vi "Xboxinterface_86.vi"() -> (2 "R Thumb":i32(slide) scale=-32768.0..32768.0)   [LabVIEW 2020]
uses:
  <vilib>/robotics/Controls/Compass Indicator/Compass Indicator.xctl
  08dc6dd9-20da-488d-be37-67a715477d84.vi
  <vilib>/Utility/inputDevices.llb/joystickAcquire.vi
  <vilib>/Utility/inputDevices.llb/closeJoystick.vi
panel:
  out "100%":bool
  out "80%":bool
  out "Analógico Direito":dbl(xcontrol)
  out "Analógico Esquerdo":dbl(xcontrol)
  out "Start":bool
  out "Stop/Back":bool
  out "Right trigger":bool
  out "Left Trigger":bool
  out "Cluster":T1
  out "LThumb":i32(slide) scale=-32768.0..32768.0
  out "Left Thumb button":bool
  out "Right Thumb button":bool
  out "LB":bool
  out "RB":bool
  out "Y":bool
  out "X":bool
  out "B":bool
  out "A":bool caption="Boolean"
  out "joystick info":T2(array[cluster])
  out "direction info":T3
  out "button info":T4
  out "axis info":T5
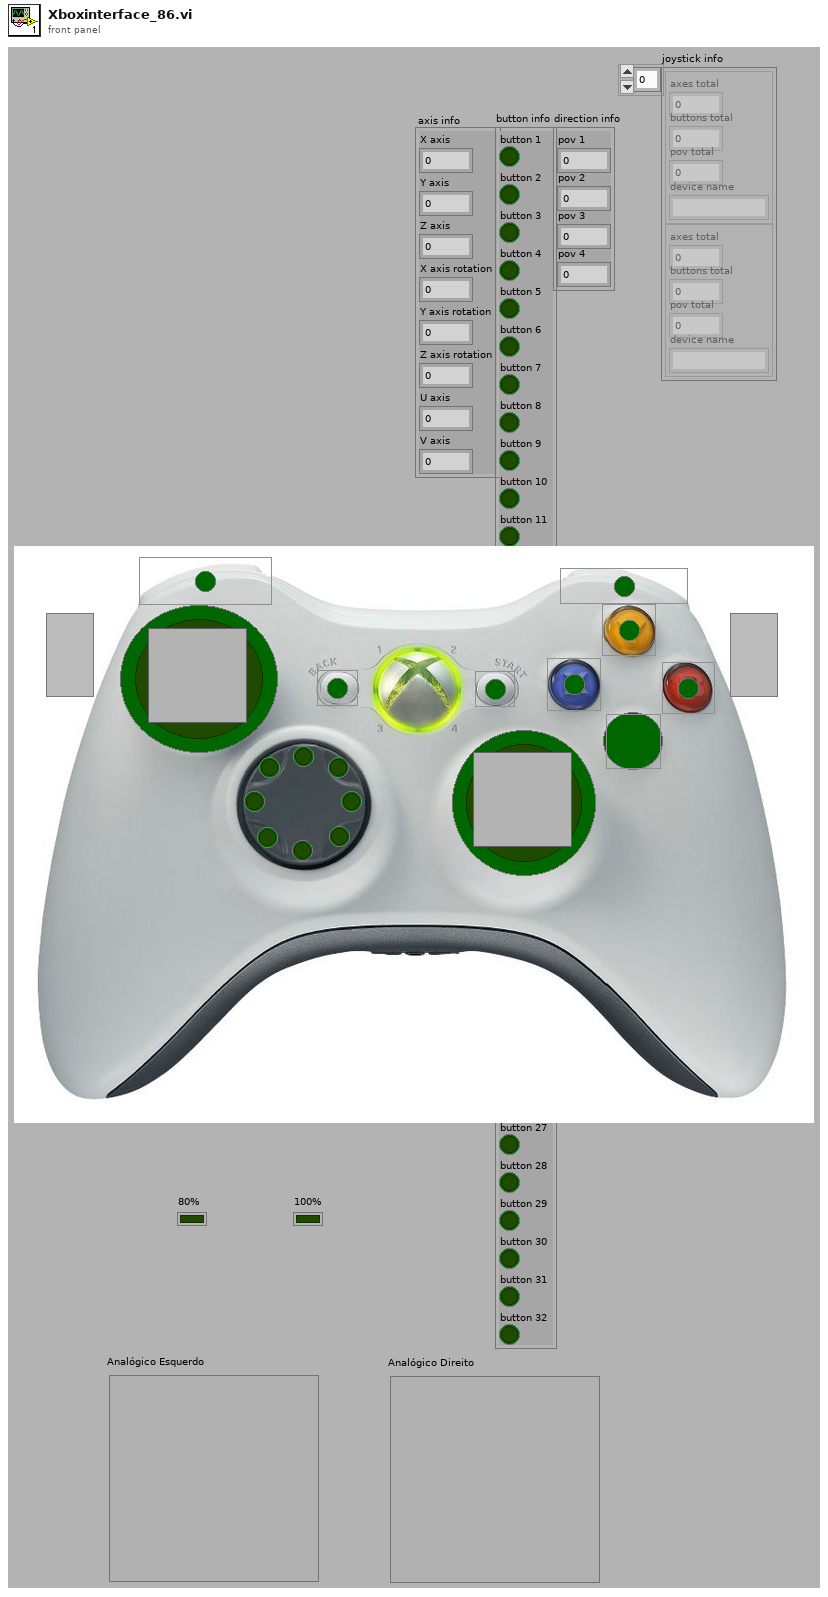
[diagram p1: front panel]
types:
  T1 = cluster{"Boolean 4":bool, "Boolean 6":bool, "Boolean 3":bool, "Boolean 7":bool, "Boolean 2":bool, "Boolean 9":bool, "Boolean 5":bool, "Boolean 8":bool}
  T2 = cluster{"axes total":u32, "buttons total":u32, "pov total":u32, "device name":string}[]
  T3 = cluster{"pov 1":i32, "pov 2":i32, "pov 3":i32, "pov 4":i32}
  T4 = cluster{"button 1":bool, "button 2":bool, "button 3":bool, "button 4":bool, "button 5":bool, "button 6":bool, "button 7":bool, "button 8":bool, "button 9":bool, "button 10":bool, "button 11":bool, "button 12":bool, "button 13":bool, "button 14":bool, "button 15":bool, "button 16":bool, "button 17":bool, "button 18":bool, "button 19":bool, "button 20":bool, "button 21":bool, "button 22":bool, "button 23":bool, "button 24":bool, "button 25":bool, "button 26":bool, "button 27":bool, "button 28":bool, "button 29":bool, "button 30":bool, "button 31":bool, "button 32":bool}
  T5 = cluster{"X axis":i32, "Y axis":i32, "Z axis":i32, "X axis rotation":i32, "Y axis rotation":i32, "Z axis rotation":i32, "U axis":i32, "V axis":i32}
  T6 = cluster{"Array[0]":bool, "Array[1]":bool, "Array[2]":bool, "Array[3]":bool, "Array[4]":bool, "Array[5]":bool, "Array[6]":bool, "Array[7]":bool}
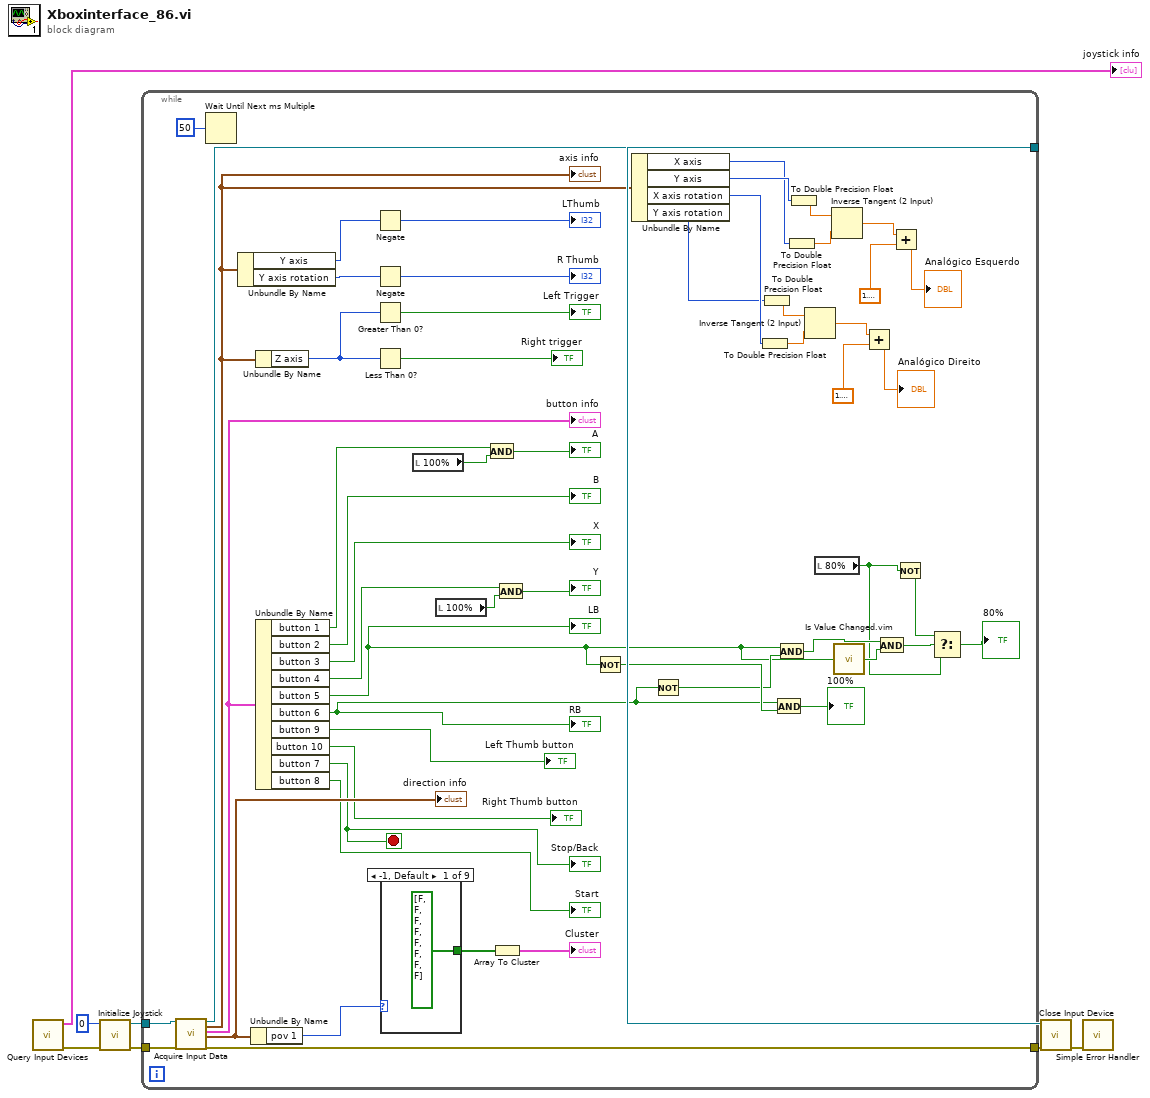
[diagram p0: block diagram]
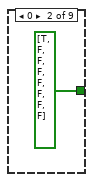
[diagram p2: hidden frame]
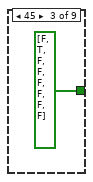
[diagram p3: hidden frame]
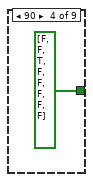
[diagram p4: hidden frame]
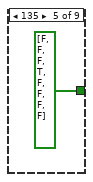
[diagram p5: hidden frame]
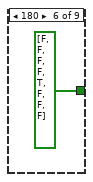
[diagram p6: hidden frame]
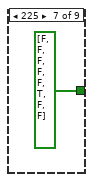
[diagram p7: hidden frame]
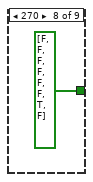
[diagram p8: hidden frame]
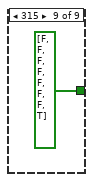
[diagram p9: hidden frame]
diagram:
  n1 = call <vilib>:"Query Input Devices.vi"() -> ("error out"=w2:errorcluster, "joystick info"=→"joystick info":T2)  [unwired: 1 in, 9 out]
  n2 = call <vilib>:"Initialize Joystick.vi"("error in (no error)"=w2, "device index"=0) -> ("error out"=w6:errorcluster, "device ID"=w7:refnum<k1>)  [unwired: 8 out]
  n3 = while {
    tunnel: w7 -> [w63]
    tunnel: w6 -> [w62]
    tunnel: [w61] -> w5
    tunnel: [w47] -> w4
    stop <- w45 stop-if-true
    n4 = call-poly <vilib>:"Acquire Input Data.vi"("device ID"=w63, "error in (no error)"=w62) -> ("device ID"=w61:refnum<k1>, "axis info"=w37:T5, "button info"=w60:T4, "direction info"=w56:T3, "error out"=w47:errorcluster)  [unwired: 13 out]
    "axis info" <- w37
    "button info" <- w60
    "direction info" <- w56
    n5 = Wait Until Next ms Multiple(millisecond multiple=u32 50) -> ()  [unwired: 1 out]
    n6 = Unbundle By Name(w37) -> ("Y axis"=w42:i32, "Y axis rotation"=w57:i32)
    n7 = Unbundle By Name(w56) -> ("pov 1"=w55:i32)
    n8 = Unbundle By Name(w37) -> ("Z axis"=w50:i32)
    n9 = Unbundle By Name(w60) -> ("button 1"=w21:bool, "button 2"=→"B":bool, "button 3"=→"X":bool, "button 4"=w17:bool, "button 5"=w14:bool, "button 6"=w25:bool, "button 9"=→"Left Thumb button":bool, "button 10"=→"Right Thumb button":bool, "button 7"=w45:bool, "button 8"=→"Start":bool)
    "RB" <- w25
    "LB" <- w14
    "Stop/Back" <- w45
    n10 = Negate(x=w42) -> (-x=→"LThumb":i32)
    n11 = Negate(x=w57) -> (-x=→"R Thumb":i32)
    n12 = Greater Than 0?(x=w50) -> (x > 0?=→"Left Trigger":bool)
    n13 = Less Than 0?(x=w50) -> (x < 0?=→"Right trigger":bool)
    n14 = case shown="-1, Default" w55 {
      tunnel: [bool[] [FALSE, FALSE, FALSE, FALSE, FALSE, FALSE, FALSE, FALSE] ("Array") bool[] [TRUE, FALSE, FALSE, FALSE, FALSE, FALSE, FALSE, FALSE] ("Array") bool[] [FALSE, TRUE, FALSE, FALSE, FALSE, FALSE, FALSE, FALSE] ("Array") bool[] [FALSE, FALSE, TRUE, FALSE, FALSE, FALSE, FALSE, FALSE] ("Array") bool[] [FALSE, FALSE, FALSE, TRUE, FALSE, FALSE, FALSE, FALSE] ("Array") bool[] [FALSE, FALSE, FALSE, FALSE, TRUE, FALSE, FALSE, FALSE] ("Array") bool[] [FALSE, FALSE, FALSE, FALSE, FALSE, TRUE, FALSE, FALSE] ("Array") bool[] [FALSE, FALSE, FALSE, FALSE, FALSE, FALSE, TRUE, FALSE] ("Array") bool[] [FALSE, FALSE, FALSE, FALSE, FALSE, FALSE, FALSE, TRUE] ("Array")] -> w54
      frame -1, Default {
      }
      frame 0 {
      }
      frame 45 {
      }
      frame 90 {
      }
      frame 135 {
      }
      frame 180 {
      }
      frame 225 {
      }
      frame 270 {
      }
      frame 315 {
      }
    }
    n15 = local read "100%"() -> (w20:bool)
    n16 = local read "100%"() -> (w18:bool)
    n17 = And(x=w21, y=w20) -> (x .and. y?=→"A":bool)
    n18 = Array To Cluster(array=w54) -> (cluster=→"Cluster":T6)
    n19 = And(x=w17, y=w18) -> (x .and. y?=→"Y":bool)
    n20 = Not(x=w14) -> (.not. x?=w26:bool)
    n21 = Unbundle By Name(w37) -> ("X axis"=w23:i32, "Y axis"=w40:i32, "X axis rotation"=w28:i32, "Y axis rotation"=w27:i32)
    n22 = Not(x=w25) -> (.not. x?=w24:bool)
    n23 = To Double Precision Float(number=w28) -> (double precision float=w33:dbl)
    n24 = To Double Precision Float(number=w27) -> (double precision float=w32:dbl)
    n25 = And(x=w25, y=w26) -> (x .and. y?=→"100%":bool)
    n26 = And(x=w14, y=w24) -> (x .and. y?=w13:bool)
    n27 = To Double Precision Float(number=w23) -> (double precision float=w39:dbl)
    n28 = To Double Precision Float(number=w40) -> (double precision float=w38:dbl)
    n29 = Inverse Tangent (2 Input)(1:w33, 2:w32) -> (0:w31:dbl)
    n30 = local read "80%"() -> (w9:bool)
    n31 = Inverse Tangent (2 Input)(1:w39, 2:w38) -> (0:w36:dbl)
    n32 = call "Is Value Changed.vim"("value"=w14) -> ("changed or first call?"=w15:bool)
    n33 = Add(x=w31, y=1.5707963267948966) -> (x+y=→"Analógico Direito":dbl)
    n34 = And(x=w13, y=w15) -> (x .and. y?=w12:bool)
    n35 = Add(x=w36, y=1.5707963267948966) -> (x+y=→"Analógico Esquerdo":dbl)
    n36 = Not(x=w9) -> (.not. x?=w11:bool)
    n37 = Select(t=w11, s=w12, f=w9) -> (s? t:f=→"80%":bool)
  }
  n38 = call-poly <vilib>:"Close Input Device.vi"("error in (no error)"=w4, "device ID"=w5) -> ("error out"=w1:errorcluster)  [unwired: 8 out]
  n39 = call <vilib>:"Simple Error Handler.vi"("error in (no error)"=w1) -> ()  [unwired: 1 in, 8 out]
